vi "HENES_Arduino_Main.vi"() -> ()   [LabVIEW 2023]
uses:
  <vilib>/Instr/_visa.llb/VISA Set IO Buffer Mask.ctl
  <vilib>/Instr/_visa.llb/VISA Flush IO Buffer Mask.ctl
  <vilib>/Platform/TimedLoop/XDataNode/timing_clust.ctl
  <vilib>/Platform/TimedLoop/XDataNode/nitl_modes.ctl
  <vilib>/Platform/TimedLoop/XDataNode/wakeup.ctl
  0e367d9d-ada3-461a-9650-c8cddcce4376.vi
  <vilib>/Utility/file.llb/Read Delimited Spreadsheet (DBL).vi
  <vilib>/Utility/file.llb/Write Delimited Spreadsheet (string).vi
  <vilib>/Instr/_visa.llb/VISA Configure Serial Port (Instr).vi
  <vilib>/Analysis/geometry.llb/Point in Polygon (Array).vi
  <vilib>/Platform/TimedLoop/XDataNode/XDataNode.xnode
  <vilib>/Platform/TimedLoop/XDataNode/XDNodeRunTimeDep.lvlib
  <vilib>/Analysis/NI_AAL_Geometry.lvlib
panel:
  out "read buffer":string
  out "Loop Time":u32=102
  out "배열":dbl[](array[numeric])
  in  "탭 컨트롤":enum32{"Main", "GPS", "ETC."}(tab)
  out "강제 변환(x)":i16
  in  "링":u16(ring) items=["정사각형ROI", "삼각형ROI"]
  in  "ROI_Y":i32=800
  in  "ROI_X":i32=200
  in  "격자크기":dbl=20.0
  out "GO?":bool
  out "Steer_CMD(Deg)":dbl
  out "UTM X(E) INS":dbl format="%#_13g"
  out "UTM Y(N) INS":dbl format="%#_13g"
  out "Near Point":i32
  out "Tracking_Err(m)":dbl
  in  "HLV_Gear":u8
  in  "HLV_A/M":bool
  in  "Input_Spd(kph)":dbl
  out "Remote_M/A":bool
  out "E-STOP":bool
  in  "Map Refresh":bool
  in  "RDDF":path=path "경로를 입력하세요."
  out "Steer_Feed":dbl
  out "Gear_Feed":u8
  out "XY Graph":T1(graph)
  in  "LOG_Forder":path=path "경로를 입력하세요."
  in  "Data Save On/Off":bool
  in  "COM4":refnum<visa-resource-name>="COM18" caption="GPS_Com."
  in  "COM5":refnum<visa-resource-name>="COM16" caption="HENES_Com."
  out "LiDAR_ROI":cluster{"X좌표":i32[], "Y좌표":i32[]}[](graph)
  in  "COM4 2":refnum<visa-resource-name>="COM16" caption="LiDAR_Com."
  out "Alive_PCU":u8(slide) scale=0.0..254.0
  out "GPS_Speed(kph)":dbl format="%#_g kph"
  out "Speed_Feed(RPM)":dbl format="%#_g rpm"
  out "True_Heading":dbl format="%#_15g"
  out "Evt":dbl
  out "WP_no.":i32
  out "Y_long_path_Full":dbl[](array[numeric])
  out "vel. path":dbl[](array[numeric])
  out "X_lat_path_Full":dbl[](array[numeric])
  out "Path_Evt_arr":dbl[](array[numeric])
  out "Path_Vel_arr":dbl[](array[numeric])
  out "Path_long_arr":dbl[](array[numeric])
  out "Path_lat_arr":dbl[](array[numeric])
  out "Evt.Arr":dbl[](array[numeric])
  out "NMEA_Raw_Data":string
  out "RDDF_Velocity":dbl
  out "Output_Spd_CMD(%)":dbl
  out "Size_init":i32
  out "Output_Spd_CMD(kph)":dbl
  in  "Stop":bool
  # "HENES Autonomous Program"
  # "※ 본 프로그램은 무료 배포 프로그램으로 상업용으로는 사용하지 말 것이며 사용 시 생기는 문제에 대해서 작성자는 책임지지 않습니다."
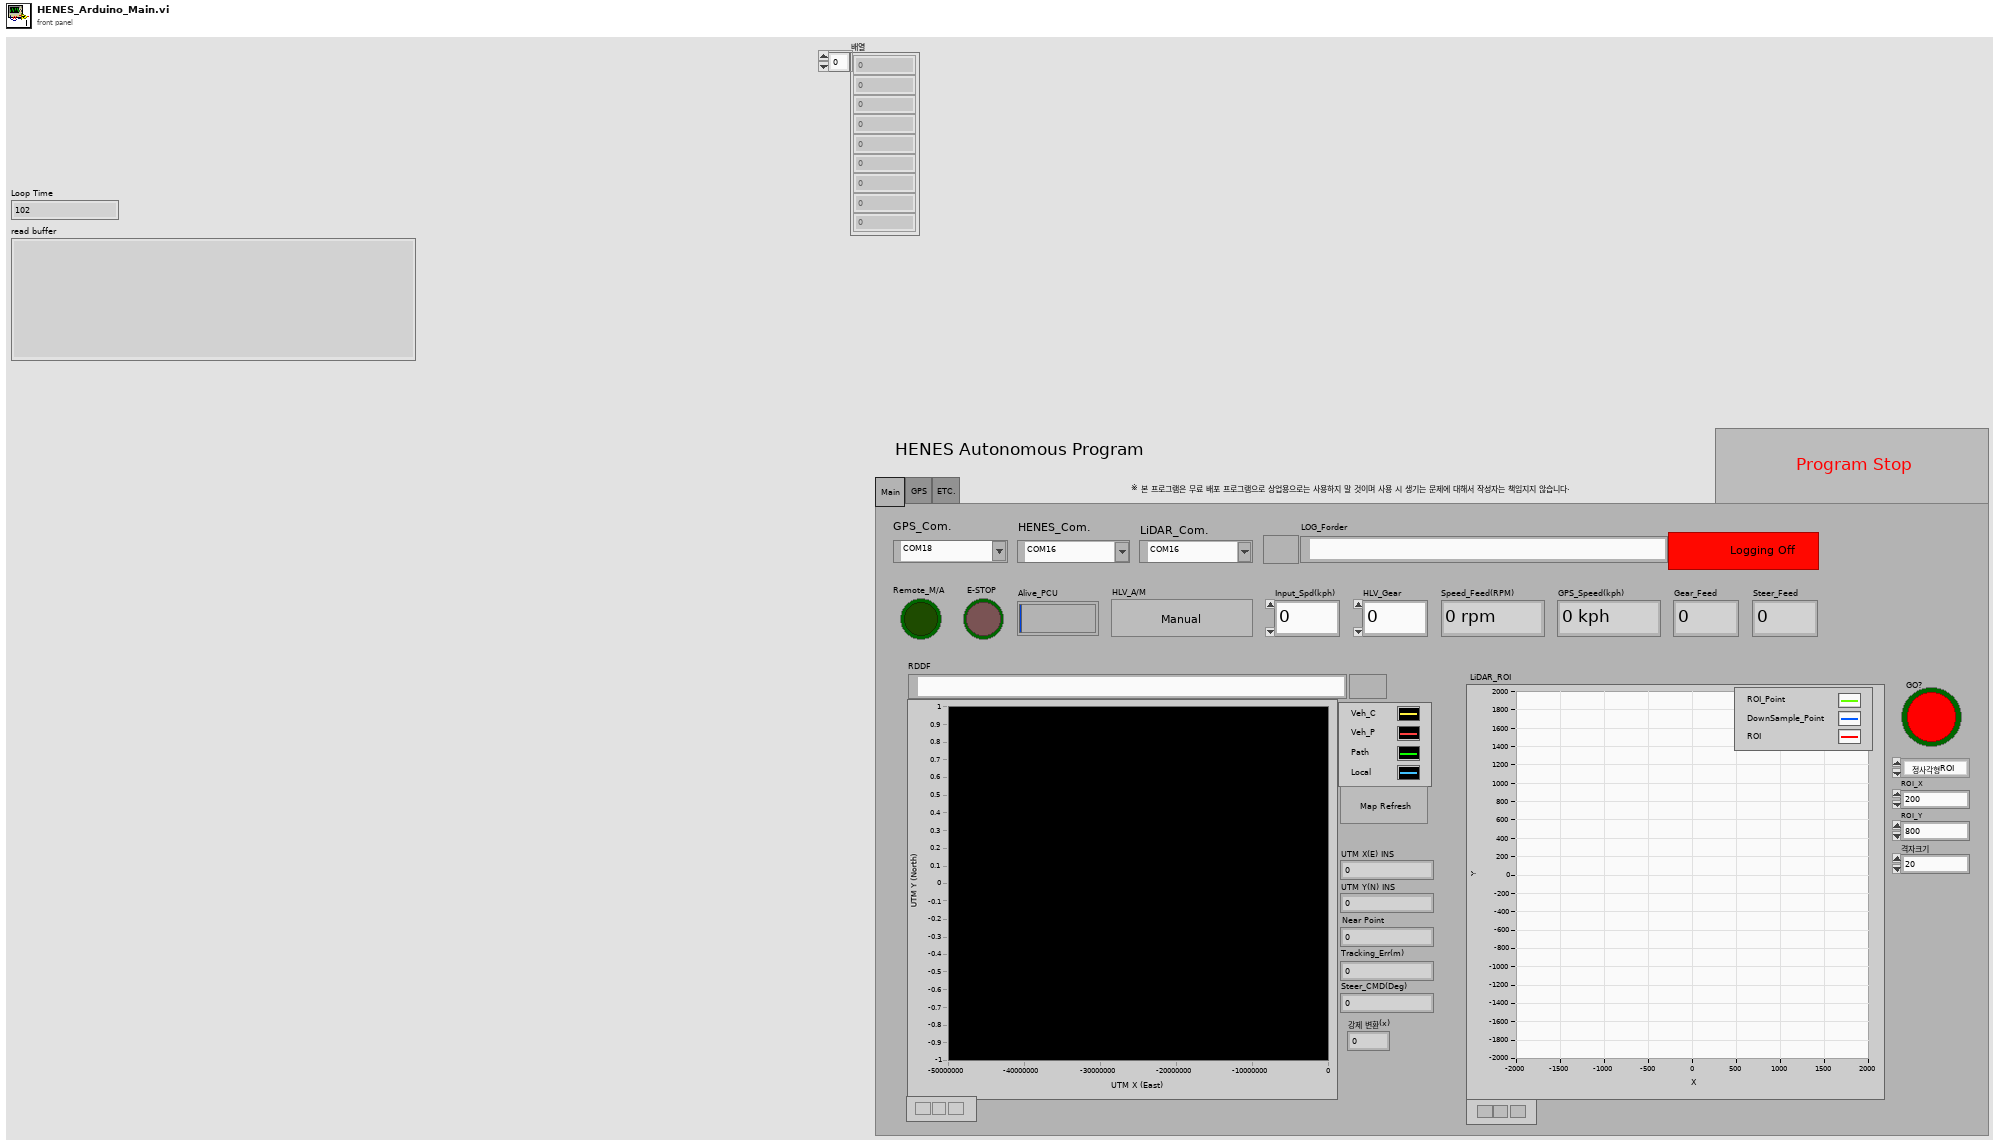
[diagram p1: front panel]
types:
  T1 = cluster{"y_long_path":dbl[], "x_lat_path":dbl[]}[]
  T2 = typedef "VISA Flush IO Buffer Mask.ctl" = u16
  T3 = typedef "VISA Set IO Buffer Mask.ctl" = u16
  T4 = cluster{"HENES_Speed":i16, "HENES_Steer":i16, "HENES_Gear":u8, "HENES_Alive":u8}
  T5 = cluster{"HLV_M/A_Status":u8, "HLV_Speed":i16, "HLV_Steer":i16, "HLV_Gear":u8, "HLV_E-Stop":u8, "HLV_Alive":u8}
  T6 = cluster{"oldest read timestamp":dbl, "latitude (deg)":dbl, "longitude (deg)":dbl, "ground speed (kph)":dbl, "true track angle (deg)":dbl, "altitude above mean sea level (m)":dbl}
  T7 = typedef "NI_AAL_Geometry.lvlib/Point in Polygon Position.ctl" = u16
  T8 = typedef "XDNodeRunTimeDep.lvlib/timing_clust.ctl" = cluster{"Expected End [f-1]":u64, "Actual End [f-1]":u64, "Finished Late? [f-1]":bool, "Expected End [i-1]":u64, "Actual End [i-1]":u64, "Finished Late? [i-1]":bool, "Expected Start [i]":u64, "Actual Start [i]":u64, "Expected Start [f]":u64, "Actual Start [f]":u64, "Source Name":string, "Structure Name":string, "Period":i64, "Deadline":i64, "Offset":i64, "Start":i64, "Priority":i32, "Timeout":i32, "Mode":T9, "Wakeup Reason":T10, "Error":errorcluster, "Source Type":string, "Secondary Source Type":string, "Global End Time":u64, "Global Start Time":u64, "Frame Duration":u64, "Iteration Duration":u64, "Assigned CPU":i32, "I/O Scan Engine Mode":u32}
  T9 = typedef "XDNodeRunTimeDep.lvlib/nitl_modes.ctl" = enum32{"No Change", "Process missed periods, maintain original phase", "Discard missed periods, maintain original phase", "Process missed periods, ignore original phase", "Discard missed periods, ignore original phase"}
  T10 = typedef "XDNodeRunTimeDep.lvlib/wakeup.ctl" = enum32{"Normal", "Aborted", "Asynchronous wakeup", "Timing source error", "Timed loop error", "Timeout"}
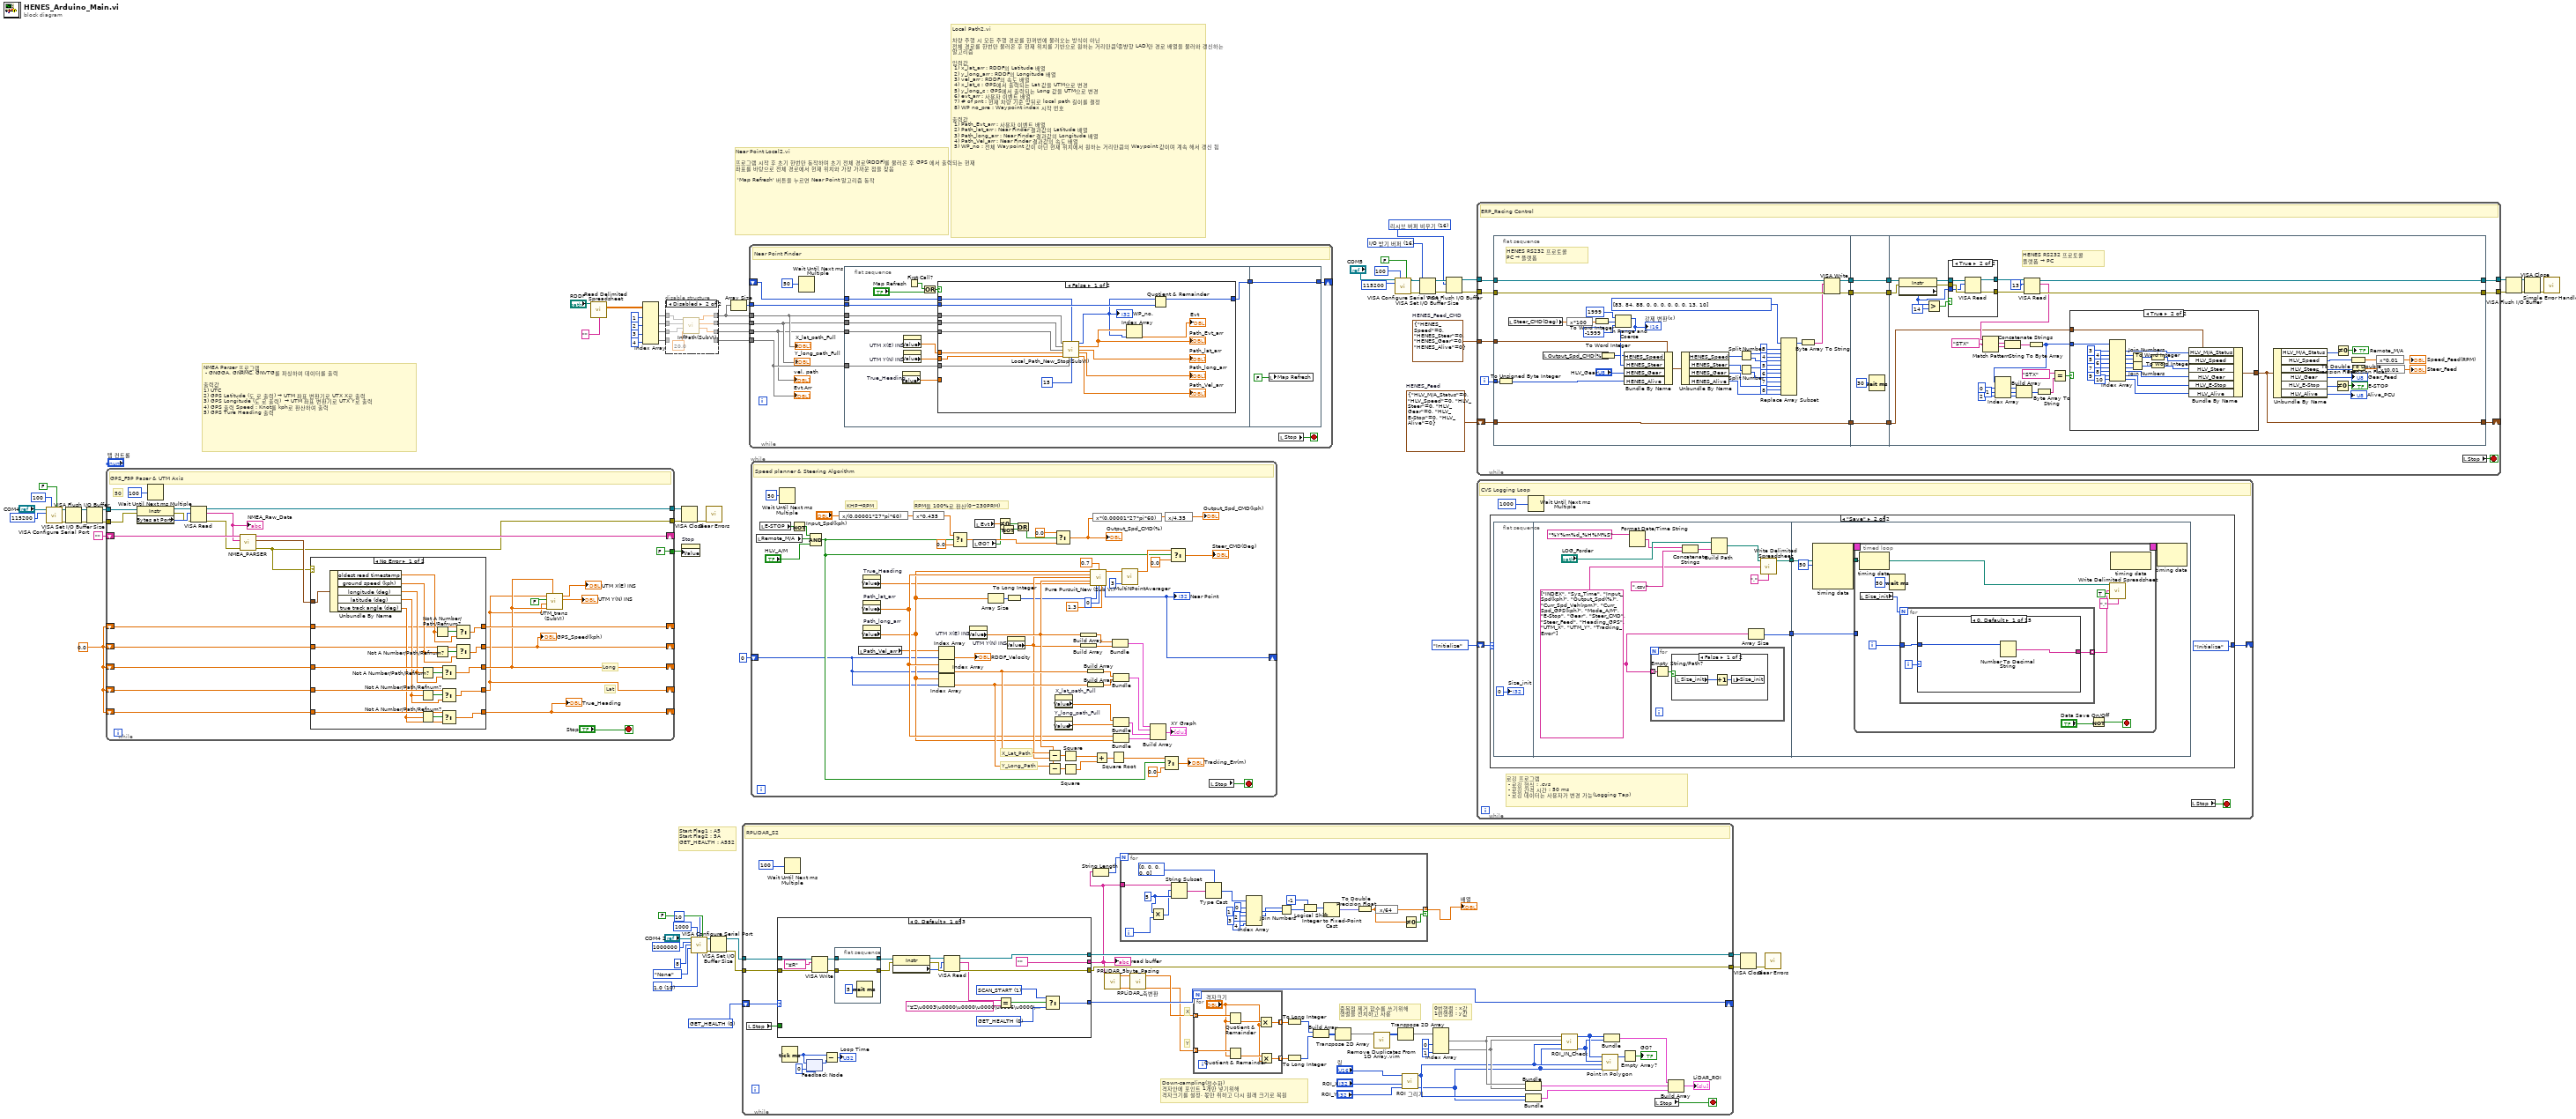
[diagram p0: block diagram]
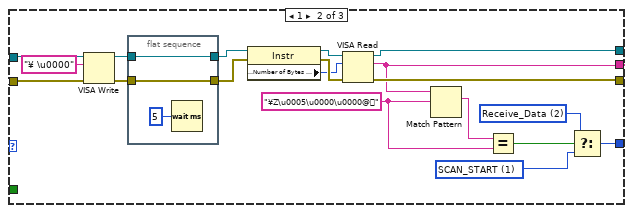
[diagram p2: hidden frame]
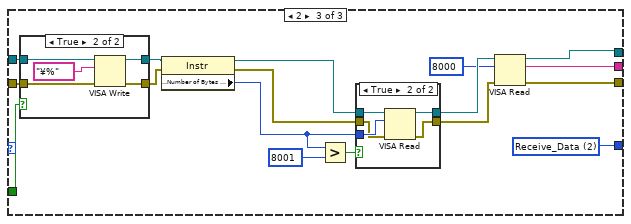
[diagram p3: hidden frame]
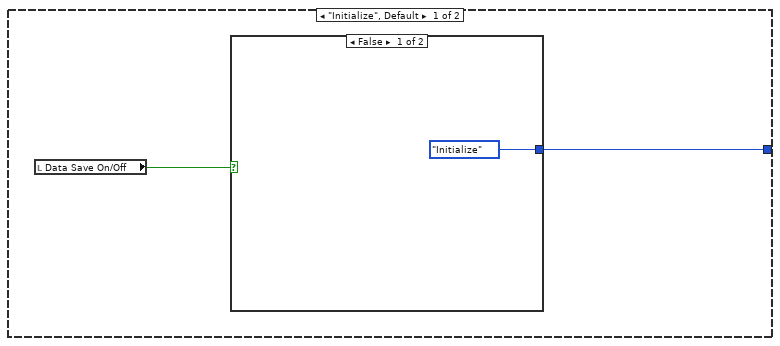
[diagram p6: hidden frame]
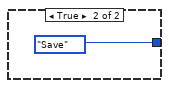
[diagram p7: hidden frame]
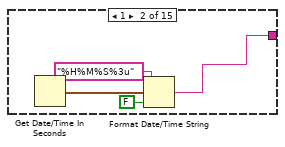
[diagram p9: hidden frame]
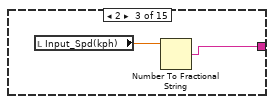
[diagram p10: hidden frame]
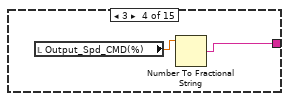
[diagram p11: hidden frame]
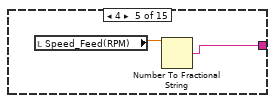
[diagram p12: hidden frame]
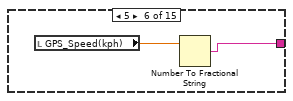
[diagram p13: hidden frame]
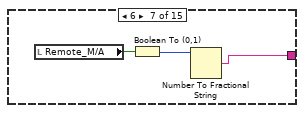
[diagram p14: hidden frame]
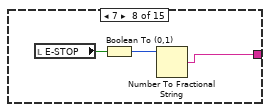
[diagram p15: hidden frame]
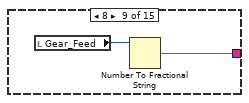
[diagram p16: hidden frame]
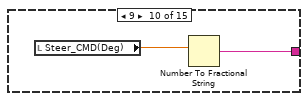
[diagram p17: hidden frame]
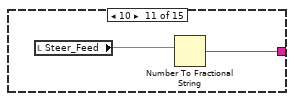
[diagram p18: hidden frame]
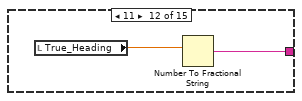
[diagram p19: hidden frame]
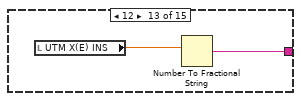
[diagram p20: hidden frame]
diagram:
  w3 = T2 16 items=["리시브 버퍼 비우기"=16, "전달 버퍼 디바이스에 쓰기"=32, "리시브 버퍼 비우기(I/O 없음)"=64, "전달 버퍼 비우기"=128] ("Mask")
  w6 = T3 16 items=["I/O 받기 버퍼"=16, "I/O 전달 버퍼"=32, "I/O 받기와 전달 버퍼"=48] ("Mask")
  w17 = u16 10 items=["1.0"=10, "1.5"=15, "2.0"=20] ("stop bits (10: 1 bit)")
  w19 = u16 0 items=["GET_HEALTH", "SCAN_START", "Receive_Data"]
  w35 = T4 {"HENES_Speed"=0, "HENES_Steer"=0, "HENES_Gear"=0, "HENES_Alive"=0}  # HENES_Feed_CMD
  w34 = T5 {"HLV_M/A_Status"=0, "HLV_Speed"=0, "HLV_Steer"=0, "HLV_Gear"=0, "HLV_E-Stop"=0, "HLV_Alive"=0}  # HENES_Feed
  w54 = 0.0 ("x")
  # "Start Flag1 : A5\nStart Flag2 : 5A \nGET_HEALTH : A552"
  # "NMEA Parser 프로그램\n - GNGGA, GNRMC, GNVTG를 파싱하여 데이터를 출력\n\n출력값 \n1) UTC\n2) GPS Latitude (도 로 출력) → UTM 좌표 변환기로 UTX X로 출력\n3) GPS Longitude (도 로 출력)  → UTM 좌표 변환기로 UTX Y로 출력\n4) GPS 출력 Speed : Knot를 kph로 환산하여 출력\n5) GPS Ture Heading 출력"
  # "Near Point Local2.vi\n\n프로그램 시작 후 초기 한번만 동작하며 초기 전체 경로(RDDF)를 불러온 후 GPS 에서 출력되는 현재 좌표를 바탕으로 전체 경로에서 현재 위치와 가장 가까운 점을 찾음\n\n 'Map Refresh' 버튼을 누르면 Near Point 알고리즘 동작"
  # "Local Path2.vi\n\n차량 주행 시 모든 주행 경로를 한꺼번에 불러오는 방식이 아닌\n전체 경로를 한번만 불러온 후 현재 위치를 기반으로 원하는 거리만큼(종뱡항 LAD)만 경로 배열을 불러와 갱신하는 알고리즘\n\n입력값 \n 1) x_lat_arr : RDDF의 Latitude 배열\n 2) y_long_arr : RDDF의 Longitude 배열\n 3) vel_arr : RDDF의 속도 배열\n 4) x_lat_c : GPS에서 출력되는 Lat 값을 UTM으로 변경\n 5) y_long_c : GPS에서 출력되는 Long 값을 UTM으로 변경\n 6) evt_arr : 사용자 이벤트 배열\n 7) # of pnt : 현재 차량 기준 앞뒤로 local path 길이를 결정\n 8) WP no_pre : Waypoint index 시작 번호\n\n출력값 \n 1) Path_Evt_arr : 사용자 이벤트 배열\n 2) Path_lat_arr : Near Finder 결과값의 Latitude 배열\n 3) Path_long_arr : Near Finder 결과값의 Longitude 배열\n 4) Path_Vel_arr : Near Finder 결과값의 속도 배열\n 5) WP_no : 전체 Waypoint 값이 아닌 현재 위치에서 원하는 거리만큼의 Waypoint 값이며 계속 해서 갱신 됨"
  n1 = call-poly "VISA Configure Serial Port"("VISA resource name"="COM4", "timeout (10sec)"=u32 100, "Enable Termination\nChar (T)"=FALSE ("Enable Termination\nChar (T)"), "baud rate (9600)"=u32 115200) -> ("VISA resource name out"=w14:refnum<visa-resource-name>, "error out"=w13:errorcluster)  [unwired: 10 in]
  n2 = VISA Set I/O Buffer Size(VISA resource name=w14, error in (no error)=w13) -> (VISA resource name out=w59:refnum<visa-resource-name>, error out=w58:errorcluster)  [unwired: 2 in]
  n3 = VISA Flush I/O Buffer(VISA resource name=w59, error in (no error)=w58) -> (VISA resource name out=w57:refnum<visa-resource-name>, error out=w56:errorcluster)  [unwired: 1 in]
  n4 = while {
    tunnel: w57 -> [w95]
    tunnel: w56 -> [w93]
    tunnel: [w97] -> w62
    tunnel: [w85] -> w60
    shift-right: [w86] -> _
    shift-left: "" -> [w90]
    shift-right: [w70] -> _
    shift-left: w54 -> [w84]
    shift-right: [w74] -> _
    shift-left: w54 -> [w83]
    shift-right: [w73] -> _
    shift-left: w54 -> [w82]
    shift-right: [w78] -> _
    shift-left: w54 -> [w81]
    shift-right: [w77] -> _
    shift-left: w54 -> [w80]
    tunnel: [FALSE] -> w53
    stop <- "Stop" stop-if-true
    # "Lat"
    # "Long"
    # "50"
    # "GPS_F9P Paser & UTM Axis"
    n5 = property class="Instr"(reference=w95, error in=w93) -> (reference out=w94:refnum<visa-resource-name>, error out=w92:errorcluster, "Bytes at Port"=w96:u32)
    n6 = Wait Until Next ms Multiple(millisecond multiple=u32 100) -> ()  [unwired: 1 out]
    n7 = VISA Read(VISA resource name=w94, byte count=w96, error in (no error)=w92) -> (VISA resource name out=w97:refnum<visa-resource-name>, read buffer=w89:string, error out=w87:errorcluster)  [unwired: 1 out]
    "NMEA_Raw_Data" <- w89
    n8 = call "NMEA_PARSER.vi"("previous partial sentence"=w90, "sensor data"=w89, "error in (no error)"=w87) -> ("remaining partial sentence"=w86:string, "GPS data"=w88:T6, "error out"=w85:errorcluster)  [unwired: 5 in]
    n9 = case shown="No Error" w85 {
      tunnel: w88 -> [w118 _]
      tunnel: w83 -> [w114 w123]
      tunnel: w82 -> [w113 w122]
      tunnel: w81 -> [w112 w121]
      tunnel: [w108 w123] -> w74
      tunnel: [w107 w122] -> w73
      tunnel: [w106 w121] -> w78
      tunnel: w84 -> [w103 w120]
      tunnel: [w102 w120] -> w70
      tunnel: w80 -> [w99 w119]
      tunnel: [w98 w119] -> w77
      frame No Error {
        n10 = Unbundle By Name(w118) -> ("oldest read timestamp"=w100:dbl, "ground speed (kph)"=w104:dbl, "longitude (deg)"=w111:dbl, "latitude (deg)"=w110:dbl, "true track angle (deg)"=w109:dbl)
        n11 = Not A Number/Path/Refnum?(number/path/refnum=w111) -> (NaN/Path/Refnum?=w117:bool)
        n12 = Not A Number/Path/Refnum?(number/path/refnum=w110) -> (NaN/Path/Refnum?=w116:bool)
        n13 = Not A Number/Path/Refnum?(number/path/refnum=w109) -> (NaN/Path/Refnum?=w115:bool)
        n14 = Not A Number/Path/Refnum?(number/path/refnum=w100) -> (NaN/Path/Refnum?=w101:bool)
        n15 = Not A Number/Path/Refnum?(number/path/refnum=w104) -> (NaN/Path/Refnum?=w105:bool)
        n16 = Select(t=w114, s=w117, f=w111) -> (s? t:f=w108:dbl)
        n17 = Select(t=w113, s=w116, f=w110) -> (s? t:f=w107:dbl)
        n18 = Select(t=w112, s=w115, f=w109) -> (s? t:f=w106:dbl)
        n19 = Select(t=w99, s=w101, f=w100) -> (s? t:f=w98:dbl)
        n20 = Select(t=w103, s=w105, f=w104) -> (s? t:f=w102:dbl)
      }
      frame Error {
        # "Invalid data points."
      }
    }
    "True_Heading" <- w78
    "GPS_Speed(kph)" <- w70
    n21 = call "UTM_trans (SubVI).vi"("Long_Deg"=w74, "long"=w74, "lat"=w73, "East?West?"=FALSE, "Lat_Deg"=w73) -> ("UTM_Y(Northing)"=→"UTM Y(N) INS":dbl, "UTM_X(Easting)"=→"UTM X(E) INS":dbl)  [unwired: 2 out]
  }
  n22 = call-poly <vilib>:"Read Delimited Spreadsheet.vi"("file path (dialog if empty)"="RDDF", "delimiter (\\t)"="" ("delimiter (\\t)")) -> ("all rows"=w64:dbl[][])  [unwired: 8 in, 5 out]
  n23 = Index Array(array=w64, index (col) #1=1 ("비활성화된 인덱스 (열)"), index (col) #2=2 ("인덱스 (열)"), index (col) #3=3 ("인덱스 (열)"), index (col) #4=4 ("인덱스 (열)")) -> (element #1=w43:dbl[], element #2=w42:dbl[], element #3=w41:dbl[], element #4=w40:dbl[])  [unwired: 4 in]
  n24 = disable-structure shown="Disabled" {
    disable-tunnel: w43 -> [w127 w134]
    disable-tunnel: w42 -> [w126 w133]
    disable-tunnel: w41 -> [w125 w132]
    disable-tunnel: w40 -> [w124 _]
    disable-tunnel: [w127 w130] -> w39
    disable-tunnel: [w126 w129] -> w38
    disable-tunnel: [w125 w128] -> w37
    disable-tunnel: [w124 _] -> w36
    frame Enabled {
    }
    frame Disabled {
      n25 = call "InfPath(SubVI).vi"("Mod dist."=20.0, "vel."=w132, "y_long"=w133, "x_lat"=w134) -> ("vel. path"=w128:dbl[], "y_long_path"=w129:dbl[], "x_lat_path"=w130:dbl[])  [unwired: 1 out]
    }
  }
  n26 = VISA Close(VISA resource name=w62, error in (no error)=w60) -> (error out=w61:errorcluster)
  n27 = property on="Stop" class="Bool (strict)"("Value"=w53) -> ()  [unwired: 2 in, 2 out]
  n28 = call-poly "VISA Configure Serial Port"("VISA resource name"="COM4 2", "timeout (10sec)"=u32 1000, "termination char\n(0xA = '\\n' = LF)"=u8 10 ("termination char\n(0xA = '\\n' = LF)"), "Enable Termination\nChar (T)"=FALSE ("Enable Termination\nChar (T)"), "baud rate (9600)"=u32 1000000, "data bits (8)"=u16 8, "parity (0:none)"=enum16{"None", "Odd", "Even", "Mark", "Space"}."None", "stop bits (10: 1 bit)"=w17) -> ("VISA resource name out"=w27:refnum<visa-resource-name>, "error out"=w26:errorcluster)  [unwired: 6 in]
  n29 = call <vilib>:"Clear Errors.vi"("error in (no error)"=w61) -> ()  [unwired: 5 in, 2 out]
  n30 = VISA Set I/O Buffer Size(VISA resource name=w27, error in (no error)=w26) -> (VISA resource name out=w21:refnum<visa-resource-name>, error out=w20:errorcluster)  [unwired: 2 in]
  n31 = Array Size(array=w39) -> (size(s)=w66:i32)
  n32 = while {
    tunnel: [w169] -> w31
    tunnel: [w170] -> w30
    tunnel: w21 -> [w178]
    tunnel: w20 -> [w177]
    shift-right: [w176] -> _
    shift-left: w19 -> [w179]
    stop <- w135 stop-if-true
    # "0번행렬 : x값\n1번행렬 : y값"
    # "중복점 제거 함수를 쓰기위해\n행렬을 전치하고 사용"
    # "Down-sampling(정수화)\n격자안에 포인트 1개만 넣기위해\n격자크기를 설정, 몫만 취하고 다시 원래 크기로 복원"
    # "Y"
    # "X"
    # "RPLIDAR_S2"
    n33 = local read "Stop"() -> (w175:bool)
    n34 = case shown="0, Default" w179 {
      tunnel: w178 -> [w225 w243 w266]
      tunnel: w177 -> [w224 w242 w265]
      tunnel: [w226 w239 w252] -> w176
      tunnel: [w215 w240 w268] -> w170
      tunnel: [w214 w241 w267] -> w169
      tunnel: w175 -> [_ _ w264]
      tunnel: ["" ("read buffer") w237 w263] -> w137
      frame 0, Default {
        w208 = u16 0 items=["GET_HEALTH", "SCAN_START", "Receive_Data"]
        w209 = u16 1 items=["GET_HEALTH", "SCAN_START", "Receive_Data"]
        n35 = VISA Write(VISA resource name=w225, write buffer="¥R", error in (no error)=w224) -> (VISA resource name out=w219:refnum<visa-resource-name>, error out=w218:errorcluster)  [unwired: 1 out]
        n36 = flat-sequence {
          tunnel: w219 -> [w228]
          tunnel: w218 -> [w227]
          tunnel: [w228] -> w217
          tunnel: [w227] -> w216
          frame #0 {
            n37 = Wait (ms)(milliseconds to wait=u32 5 ("대기 시간 (ms)")) -> ()  [unwired: 1 out]
          }
        }
        n38 = property class="Instr"(reference=w217, error in=w216) -> (reference out=w222:refnum<visa-resource-name>, error out=w221:errorcluster, "Serial Settings:Number of Bytes at Serial Port"=w220:u32)
        n39 = VISA Read(VISA resource name=w222, byte count=w220, error in (no error)=w221) -> (VISA resource name out=w214:refnum<visa-resource-name>, read buffer=w211:string, error out=w215:errorcluster)  [unwired: 1 out]
        n40 = Equal?(x=w211, y="¥Z\u0003\u0000\u0000\u0000\u0006\u0000\u0000\u0000") -> (x = y?=w212:bool)
        n41 = Select(t=w209, s=w212, f=w208) -> (s? t:f=w226:u16)
      }
      frame 1 {
        w230 = u16 2 items=["GET_HEALTH", "SCAN_START", "Receive_Data"]
        w231 = u16 1 items=["GET_HEALTH", "SCAN_START", "Receive_Data"]
        w244 = "¥Z\u0005\u0000\u0000@"
        n42 = VISA Write(VISA resource name=w243, write buffer="¥ \u0000", error in (no error)=w242) -> (VISA resource name out=w246:refnum<visa-resource-name>, error out=w247:errorcluster)  [unwired: 1 out]
        n43 = flat-sequence {
          tunnel: w246 -> [w250]
          tunnel: w247 -> [w249]
          tunnel: [w250] -> w233
          tunnel: [w249] -> w232
          frame #0 {
            n44 = Wait (ms)(milliseconds to wait=u32 5 ("대기 시간 (ms)")) -> ()  [unwired: 1 out]
          }
        }
        n45 = property class="Instr"(reference=w233, error in=w232) -> (reference out=w236:refnum<visa-resource-name>, error out=w235:errorcluster, "Serial Settings:Number of Bytes at Serial Port"=w234:u32)
        n46 = VISA Read(VISA resource name=w236, byte count=w234, error in (no error)=w235) -> (VISA resource name out=w241:refnum<visa-resource-name>, read buffer=w237:string, error out=w240:errorcluster)  [unwired: 1 out]
        n47 = Match Pattern(string=w237, regular expression=w244) -> (match substring=w238:string)  [unwired: 1 in, 3 out]
        n48 = Equal?(x=w238, y=w244) -> (x = y?=w248:bool)
        n49 = Select(t=w230, s=w248, f=w231) -> (s? t:f=w239:u16)
      }
      frame 2 {
        w252 = u16 2 items=["GET_HEALTH", "SCAN_START", "Receive_Data"]
        n50 = case shown="True" w264 {
          tunnel: w266 -> [w277 w281]
          tunnel: w265 -> [w276 w280]
          tunnel: [w277 w279] -> w262
          tunnel: [w276 w278] -> w261
          frame False {
          }
          frame True {
            n51 = VISA Write(VISA resource name=w281, write buffer="¥%", error in (no error)=w280) -> (VISA resource name out=w279:refnum<visa-resource-name>, error out=w278:errorcluster)  [unwired: 1 out]
          }
        }
        n52 = property class="Instr"(reference=w262, error in=w261) -> (reference out=w257:refnum<visa-resource-name>, error out=w256:errorcluster, "Serial Settings:Number of Bytes at Serial Port"=w258:u32)
        n53 = Greater?(x=w258, y=u32 8001) -> (0:w260:bool)
        n54 = case shown="True" w260 {
          tunnel: w257 -> [w270 w275]
          tunnel: w258 -> [_ w274]
          tunnel: w256 -> [w269 w273]
          tunnel: [w270 w272] -> w255
          tunnel: [w269 w271] -> w254
          frame False {
          }
          frame True {
            n55 = VISA Read(VISA resource name=w275, byte count=w274, error in (no error)=w273) -> (VISA resource name out=w272:refnum<visa-resource-name>, error out=w271:errorcluster)  [unwired: 2 out]
          }
        }
        n56 = VISA Read(VISA resource name=w255, byte count=u32 8000, error in (no error)=w254) -> (VISA resource name out=w267:refnum<visa-resource-name>, read buffer=w263:string, error out=w268:errorcluster)  [unwired: 1 out]
      }
    }
    "read buffer" <- w137
    n57 = Tick Count (ms)() -> (millisecond timer value=w174:u32)
    n58 = Wait Until Next ms Multiple(millisecond multiple=u32 100 ("ms 배수")) -> ()  [unwired: 1 out]
    n59 = feedback #1(u32 0 ("millisecond timer value")) -> (w173:u32)
    n60 = feedback-in #1(w174) -> ()
    n61 = Subtract(x=w174, y=w173) -> (x-y=→"Loop Time":u32)
    n62 = String Length(string=w137) -> (length=w138:i32)
    n63 = call "PRLIDAR_5byte_Pasing.vi"("RPLIDAR_Data"=w137) -> ("Distance(mm)"=w150:dbl[], "Theta(deg)"=w151:dbl[])  [unwired: 9 in]
    n64 = for {
      N: w138 -> [_]
      tunnel: w137 -> [w200]
      tunnel: [w182] -> w136 mode=indexing if=w180
      i -> [w199]
      w198 = 5
      n65 = Multiply(x=w198, y=w199) -> (x*y=w197:i32)
      n66 = String Subset(string=w200, offset (0)=w197, length (rest)=w198) -> (substring=w196:string)
      n67 = Type Cast(type=u8[] [0, 0, 0, 0, 0], x=w196) -> (*(type *) &x=w194:u8[])
      n68 = Index Array(array=w194, index #1=0 ("인덱스"), index #2=1 ("인덱스"), index #3=2 ("인덱스"), index #4=3 ("인덱스"), index #5=4 ("인덱스")) -> (element #2=w188:u8, element #3=w183:u8)  [unwired: 3 out]
      n69 = Join Numbers(hi=w183, lo=w188) -> ((hi.lo)=w187:u16)
      n70 = Logical Shift(y=i16 -1, x=w187) -> (x << y=w185:u16)
      n71 = Integer to Fixed-Point Cast(integer=w185) -> (fixed-point=w184:fxp<+,16,16>)  [unwired: 1 in]
      n72 = To Double Precision Float(number=w184) -> (double precision float=w181:dbl)
      n73 = expression code="x/64"(w181) -> (w182:dbl)
      n74 = Not Equal To 0?(x=w181) -> (x != 0?=w180:bool)
    }
    "배열" <- w136
    n75 = call "RPLiDAR_축변환.vi"("Distance(mm)"=w150, "Theta(deg)"=w151) -> ("Y"=w148:dbl[], "X"=w149:dbl[])  [unwired: 8 in]
    n76 = for {
      tunnel: w149 -> [w207] mode=indexing
      tunnel: w148 -> [w206] mode=indexing
      tunnel: [w203] -> w167 mode=indexing
      tunnel: [w202] -> w168 mode=indexing
      n77 = Quotient & Remainder(x=w207, y="격자크기") -> (floor(x/y)=w205:dbl)  [unwired: 1 out]
      n78 = Quotient & Remainder(x=w206, y="격자크기") -> (floor(x/y)=w204:dbl)  [unwired: 1 out]
      n79 = Multiply(x=w205, y="격자크기") -> (x*y=w203:dbl)
      n80 = Multiply(x=w204, y="격자크기") -> (x*y=w202:dbl)
    }
    n81 = To Long Integer(number=w167) -> (32bit integer=w161:i32[])
    n82 = To Long Integer(number=w168) -> (32bit integer=w160:i32[])
    n83 = Build Array(w161, w160) -> (w163:i32[][])
    n84 = Transpose 2D Array(2D array=w163) -> (transposed array=w158:i32[][])
    n85 = call "Remove Duplicates From 1D Array.vim"("array"=w158) -> ("array with duplicates removed"=w159:i32[][])  [unwired: 10 in]
    n86 = Transpose 2D Array(2D array=w159) -> (transposed array=w164:i32[][])
    n87 = call "ROI 그리기.vi"("ROI_Y"="ROI_Y", "ROI_X"="ROI_X", "도형형태"="링") -> ("Y좌표"=w141:i32[], "X좌표"=w142:i32[])  [unwired: 7 in]
    n88 = Index Array(array=w164, index (row) #1=0 ("index (row)"), index (row) #2=1 ("index (row)")) -> (element #1=w144:i32[], element #2=w143:i32[])  [unwired: 2 in]
    n89 = Bundle(w144, w143) -> (w155:cluster{i32[], i32[]})  [unwired: 1 in]
    n90 = Bundle("X좌표"=w142, "Y좌표"=w141) -> (w154:cluster{"X좌표":i32[], "Y좌표":i32[]})  [unwired: 1 in]
    n91 = call "ROI_IN_Check.vi"("도형Y좌표"=w141, "도형X좌표"=w142, "LiDAR_Y"=w143, "LiDAR_X"=w144) -> ("ROI_IN_Y"=w139:i32[], "ROI_IN_X"=w140:i32[])  [unwired: 6 in]
    n92 = call-poly <vilib>:"Point in Polygon.vi"("Polygon Y"=w141, "Polygon X"=w142, "Y"=w139, "X"=w140) -> ("Position"=w152:T7[])  [unwired: 6 in, 1 out]
    n93 = Bundle("ROI_IN_X"=w140, "ROI_IN_Y"=w139) -> (w156:cluster{"ROI_IN_X":i32[], "ROI_IN_Y":i32[]})  [unwired: 1 in]
    n94 = Empty Array?(array=w152) -> (empty?=→"GO?":bool)
    n95 = local read "Stop"() -> (w135:bool)
    n96 = Build Array(w156, w155, w154) -> (→"LiDAR_ROI":cluster{"X좌표":i32[], "Y좌표":i32[]}[])
  }
  n97 = while {
    shift-right: [w291] -> _
    shift-left: _ -> [w292]
    tunnel: w66 -> [w289]
    tunnel: w37 -> [w283]
    tunnel: w38 -> [w284]
    tunnel: w39 -> [w285]
    tunnel: w36 -> [w288]
    stop <- w287 stop-if-true
    # "Near Point Finder"
    n98 = Wait Until Next ms Multiple(millisecond multiple=u32 50) -> ()  [unwired: 1 out]
    n99 = flat-sequence {
      tunnel: [w304] -> w290
      tunnel: w292 -> [w305]
      tunnel: w289 -> [w300]
      tunnel: w283 -> [w299]
      tunnel: w284 -> [w298]
      tunnel: w285 -> [w297]
      tunnel: w288 -> [w296]
      tunnel: [w330] -> w291
      tunnel: w290 -> [w330]
      frame #0 {
        n100 = property on="True_Heading" class="DigNum (strict)"() -> ("Value"=w293:dbl)  [unwired: 2 in, 2 out]
        n101 = property on="UTM X(E) INS" class="DigNum (strict)"() -> ("Value"=w295:dbl)  [unwired: 2 in, 2 out]
        n102 = property on="UTM Y(N) INS" class="DigNum (strict)"() -> ("Value"=w294:dbl)  [unwired: 2 in, 2 out]
        n103 = First Call?() -> (First Call?: T/F=w302:bool)
        n104 = Or(x=w302, y="Map Refresh") -> (x .or. y?=w303:bool)
        n105 = case shown="False" w303 {
          tunnel: w297 -> [w317 w328]
          tunnel: w298 -> [w318 w327]
          tunnel: w305 -> [w316 _]
          tunnel: w299 -> [w319 _]
          tunnel: w300 -> [w320 _]
          tunnel: [w321 w325] -> w304
          tunnel: w296 -> [w311 _]
          tunnel: w295 -> [w310 w324]
          tunnel: w294 -> [w309 w323]
          tunnel: w293 -> [_ w322]
          frame False {
            n106 = call "Local_Path_New_Stop(SubVI).vi"("x_lat_arr"=w317, "WP no_pre"=w316, "y_long_arr"=w318, "vel_arr"=w319, "x_lat_c"=w310, "y_long_c"=w309, "evt_arr"=w311, "# of pnt"=15) -> ("INDEX(Near Point)"=w307:i32, "Evt(Local)"=w313:dbl[], "Lat(Local)"=→"Path_lat_arr":dbl[], "Long(Local)"=→"Path_long_arr":dbl[], "Vel(Local)"=→"Path_Vel_arr":dbl[])  [unwired: 3 in]
            "WP_no." <- w307
            "Path_Evt_arr" <- w313
            n107 = Index Array(array=w313, index=w307) -> (element=→"Evt":dbl)
            n108 = Quotient & Remainder(x=w307, y=w320) -> (x-y*floor(x/y)=w321:i32)  [unwired: 1 out]
          }
          frame True {
            n109 = call "Local_Path_Second (SubVI).vi"("heading_deg"=w322, "heading_limit"=179.0, "y_long"=w323, "x_lat"=w324, "Y_long_path"=w327, "X_lat_path"=w328) -> ("Index(near vehicle)"=w325:i32)  [unwired: 1 out]
          }
        }
      }
      frame #1 {
        n110 = local write "Map Refresh"(FALSE ("Refresh")) -> ()
      }
    }
    n111 = local read "Stop"() -> (w287:bool)
    "X_lat_path_Full" <- w285
    "vel. path" <- w283
    "Y_long_path_Full" <- w284
    "Evt.Arr" <- w288
  }
  n112 = while {
    shift-right: [w375] -> _
    shift-left: 0 -> [w345]
    stop <- w355 stop-if-true
    # "RPM을 100%로 환산(0~230PRM)"
    # "KHP→RPM"
    # "X_Lat_Path"
    # "Y_Long_Path"
    # "Speed planner & Steering Algorithm"
    n113 = local read "Remote_M/A"() -> (w350:bool)
    n114 = local read "E-STOP"() -> (w346:bool)
    n115 = Wait Until Next ms Multiple(millisecond multiple=u32 50 ("ms 배수")) -> ()  [unwired: 1 out]
    n116 = Not(x=w346) -> (.not. x?=w347:bool)
    n117 = Compound Arithmetic op=AND ("복합 연산")(w347, w350, "HLV_A/M") -> (w348:bool)
    n118 = expression code="x/(0.00001*27*pi*60)"("Input_Spd(kph)") -> (w340:dbl)
    n119 = local read "Path_Vel_arr"() -> (w344:dbl[])
    n120 = property on="True_Heading" class="DigNum (strict)"() -> ("Value"=w356:dbl)  [unwired: 2 in, 2 out]
    n121 = property on="Path_lat_arr" class="Arr (strict)"() -> ("Value"=w369:dbl[])  [unwired: 2 in, 2 out]
    n122 = property on="Path_long_arr" class="Arr (strict)"() -> ("Value"=w368:dbl[])  [unwired: 2 in, 2 out]
    n123 = expression code="x*0.435"(w340) -> (w338:dbl)
    n124 = Index Array(array=w344, index=w345) -> (element=→"RDDF_Velocity":dbl)
    n125 = Index Array(array=w369, index=w345) -> (element=w384:dbl)
    n126 = Index Array(array=w368, index=w345) -> (element=w383:dbl)
    n127 = Select(t=w338, s=w348, f=0.0) -> (s? t:f=w353:dbl)
    n128 = property on="UTM X(E) INS" class="DigNum (strict)"() -> ("Value"=w373:dbl)  [unwired: 2 in, 2 out]
    n129 = local read "GO?"() -> (w332:bool)
    n130 = local read "Evt"() -> (w363:dbl)
    n131 = Array Size(array=w368) -> (size(s)=w362:i32)
    n132 = Not Equal To 0?(x=w363) -> (x != 0?=w334:bool)
    n133 = Not(x=w332) -> (.not. x?=w331:bool)
    n134 = To Long Integer(number=w362) -> (32bit integer=w361:i32)
    n135 = property on="UTM Y(N) INS" class="DigNum (strict)"() -> ("Value"=w372:dbl)  [unwired: 2 in, 2 out]
    n136 = Or(x=w334, y=w331) -> (x .or. y?=w333:bool)
    n137 = Subtract(x=w384, y=w372) -> (x-y=w382:dbl)
    n138 = Subtract(x=w383, y=w373) -> (x-y=w381:dbl)
    n139 = property on="Y_long_path_Full" class="Arr (strict)"() -> ("Value"=w370:dbl[])  [unwired: 2 in, 2 out]
    n140 = Select(t=0.0, s=w333, f=w353) -> (s? t:f=w337:dbl)
    "Output_Spd_CMD(%)" <- w337
    n141 = property on="X_lat_path_Full" class="Arr (strict)"() -> ("Value"=w371:dbl[])  [unwired: 2 in, 2 out]
    n142 = Square(x=w382) -> (x^2=w380:dbl)
    n143 = Square(x=w381) -> (x^2=w379:dbl)
    n144 = Build Array(w373) -> (w391:dbl[])
    n145 = Build Array(w372) -> (w390:dbl[])
    n146 = Build Array(w384) -> (w389:dbl[])
    n147 = Build Array(w383) -> (w388:dbl[])
    n148 = call "Pure Pursuit_New (Sub VI).vi"("x_lat_path"=w368, "L"=0.7, "y_long_path"=w369, "X_Current"=w372, "Y_Current"=w373, "Heading_Current"=w356, "#pnt"=w361, "WP no_pre"=0, "LAD"=1.3) -> ("Steer_CMD(Deg)"=w357:dbl, "Index(near vehicle)"=w375:i32)  [unwired: 3 in, 2 out]
    "Near Point" <- w375
    n149 = expression code="x*(0.00001*27*pi*60)"(w337) -> (w339:dbl)
    n150 = Add(x=w380, y=w379) -> (x+y=w378:dbl)
    n151 = Square Root(x=w378) -> (sqrt(x)=w367:dbl)
    n152 = Bundle(w391, w390) -> (w385:cluster{dbl[], dbl[]})  [unwired: 1 in]
    n153 = Bundle(w389, w388) -> (w377:cluster{dbl[], dbl[]})  [unwired: 1 in]
    n154 = Bundle("Value"=w371, "Value"=w370) -> (w386:cluster{"Value":dbl[], "Value":dbl[]})  [unwired: 1 in]
    n155 = Bundle("Value"=w369, "Value"=w368) -> (w376:cluster{"Value":dbl[], "Value":dbl[]})  [unwired: 1 in]
    n156 = call "MultiNPointAverager.vi"("N point average"=3 ("WP no_pre"), "Data_input"=w357) -> ("숫자형"=w352:dbl)  [unwired: 9 in]
    n157 = Build Array(w385, w377, w386, w376) -> (→"XY Graph":cluster{"Value":dbl[], "Value":dbl[]}[])
    n158 = Select(t=w367, s=w348, f=0.0) -> (s? t:f=→"Tracking_Err(m)":dbl)
    n159 = expression code="x/4.35"(w339) -> (→"Output_Spd_CMD(kph)":dbl)
    n160 = Select(t=w352, s=w348, f=0.0) -> (s? t:f=→"Steer_CMD(Deg)":dbl)
    n161 = local read "Stop"() -> (w355:bool)
  }
  n162 = call-poly "VISA Configure Serial Port"("VISA resource name"="COM5", "timeout (10sec)"=u32 100, "Enable Termination\nChar (T)"=FALSE ("Enable Termination\nChar (T)"), "baud rate (9600)"=u32 115200) -> ("VISA resource name out"=w2:refnum<visa-resource-name>, "error out"=w1:errorcluster)  [unwired: 10 in]
  n163 = VISA Set I/O Buffer Size(VISA resource name=w2, mask (16)=w6, error in (no error)=w1) -> (VISA resource name out=w5:refnum<visa-resource-name>, error out=w4:errorcluster)  [unwired: 1 in]
  n164 = VISA Flush I/O Buffer(VISA resource name=w5, mask (16)=w3, error in (no error)=w4) -> (VISA resource name out=w50:refnum<visa-resource-name>, error out=w49:errorcluster)
  n165 = while {
    shift-right: [w392] -> _
    shift-left: enum16{"Initialize", "Save"}."Initialize" -> [w393]
    stop <- w395 stop-if-true
    # "로깅 프로그램\n - 로깅 형식 : .cvs\n - 로깅 간격 시간 : 50 ms\n - 로깅 데이터는 사용자가 변경 가능(Logging Tap)"
    # "CVS Logging Loop"
    n166 = case shown="\"Save\"" w393 {
      tunnel: [w396 enum16{"Initialize", "Save"}."Initialize"] -> w392
      frame "Initialize", Default {
        n167 = local read "Data Save On/Off"() -> (w397:bool)
        n168 = case shown="False" w397 {
          tunnel: [enum16{"Initialize", "Save"}."Initialize" enum16{"Initialize", "Save"}."Save"] -> w396
          frame False {
          }
          frame True {
          }
        }
      }
      frame "Save" {
        n169 = flat-sequence {
          tunnel: [w412] -> w402
          tunnel: [w411] -> w401
          tunnel: w402 -> [w422]
          tunnel: w401 -> [w421]
          frame #0 {
            "Size_init" <- 0 ("Size_init")
          }
          frame #1 {
            w404 = string[] ["INDEX", "Sys_Time", "Input_Spd(kph)", "Output_Spd(%)", "Curr_Spd_Veh(rpm)", "Curr_Spd_GPS(kph)", "Mode_A/M", "E-Stop", "Gear", "Steer_CMD", "Steer_Feed", "Heading_GPS", "UTM_X", "UTM_Y", "Tracking_Error"] ("배열")
            n170 = Format Date/Time String(time format string (%c)="%Y%m%d_%H%M%S" ("시간 포맷 문자열 (%c)")) -> (date/time string=w407:string)  [unwired: 2 in]
            n171 = for {
              tunnel: w404 -> [w415] mode=indexing
              n172 = Empty String/Path?(string/path=w415) -> (empty?=w414:bool)
              n173 = case shown="False" w414 {
                frame False {
                  n174 = local read "Size_init"() -> (w417:i32)
                  n175 = Increment(x=w417) -> (x+1=w416:i32)
                  n176 = local write "Size_init"(w416) -> ()
                }
                frame True {
                }
              }
            }
            n177 = Concatenate Strings(w407, ".csv" ("string")) -> (w406:string)
            n178 = Build Path(base path="LOG_Forder", name or relative path=w406) -> (appended path=w408:path)
            n179 = Array Size(array=w404) -> (size(s)=w411:i32)
            n180 = call-poly <vilib>:"Write Delimited Spreadsheet.vi"("file path (dialog if empty)"=w408, "1D data"=w404, "delimiter (\\t)"="," ("delimiter (\\t)")) -> ("new file path (Not A Path if cancelled)"=w412:path)  [unwired: 11 in, 1 out]
          }
          frame #2 {
            n181 = node-c288(i64 50 ("Period")) -> (w420:T8)  [unwired: 3 in]
            n182 = timed-loop {
              tunnel: w422 -> [w431]
              tunnel: w421 -> [_]
              timing: w420 -> [_]
              timing-out: [_] -> w419
              i -> [w429]
              stop <- w424 stop-if-true
              n183 = node-c288() -> ()  [unwired: 1 in, 1 out]
              n184 = local read "Size_init"() -> (w426:i32)
              n185 = Wait (ms)(milliseconds to wait=u32 50) -> ()  [unwired: 1 out]
              n186 = for {
                N: w426 -> [_]
                tunnel: w429 -> [w435]
                tunnel: [w434] -> w428 mode=indexing
                i -> [w436]
                n187 = case shown="0, Default" w436 {
                  tunnel: w435 -> [w438 _ _ _ _ _ _ _ _ _ _ _ _ _ _]
                  tunnel: [w437 w439 w444 w446 w448 w450 w453 w456 w457 w459 w461 w463 w465 w468 w470] -> w434
                  frame 0, Default {
                    n188 = Number To Decimal String(number=w438) -> (decimal integer string=w437:string)  [unwired: 1 in]
                  }
                  frame 1 {
                    n189 = Get Date/Time In Seconds() -> (seconds since 1Jan1904=w441:timestamp)
                    n190 = Format Date/Time String(time format string (%c)="%H%M%S%3u", seconds (now)=w441, UTC format=FALSE) -> (date/time string=w439:string)
                  }
                  frame 2 {
                    n191 = local read "Input_Spd(kph)"() -> (w443:dbl)
                    n192 = Number To Fractional String(number=w443) -> (F-format string=w444:string)  [unwired: 3 in]
                  }
                  frame 3 {
                    n193 = local read "Output_Spd_CMD(%)"() -> (w445:dbl)
                    n194 = Number To Fractional String(number=w445) -> (F-format string=w446:string)  [unwired: 3 in]
                  }
                  frame 4 {
                    n195 = local read "Speed_Feed(RPM)"() -> (w447:dbl)
                    n196 = Number To Fractional String(number=w447) -> (F-format string=w448:string)  [unwired: 3 in]
                  }
                  frame 5 {
                    n197 = local read "GPS_Speed(kph)"() -> (w449:dbl)
                    n198 = Number To Fractional String(number=w449) -> (F-format string=w450:string)  [unwired: 3 in]
                  }
                  frame 6 {
                    n199 = local read "Remote_M/A"() -> (w451:bool)
                    n200 = Boolean To (0,1)(Boolean=w451) -> (0, 1=w452:i16)
                    n201 = Number To Fractional String(number=w452) -> (F-format string=w453:string)  [unwired: 3 in]
                  }
                  frame 7 {
                    n202 = local read "E-STOP"() -> (w455:bool)
                    n203 = Boolean To (0,1)(Boolean=w455) -> (0, 1=w454:i16)
                    n204 = Number To Fractional String(number=w454) -> (F-format string=w456:string)  [unwired: 3 in]
                  }
                  frame 8 {
                    n205 = local read "Gear_Feed"() -> (w458:u8)
                    n206 = Number To Fractional String(number=w458) -> (F-format string=w457:string)  [unwired: 3 in]
                  }
                  frame 9 {
                    n207 = local read "Steer_CMD(Deg)"() -> (w460:dbl)
                    n208 = Number To Fractional String(number=w460) -> (F-format string=w459:string)  [unwired: 3 in]
                  }
                  frame 10 {
                    n209 = local read "Steer_Feed"() -> (w462:dbl)
                    n210 = Number To Fractional String(number=w462) -> (F-format string=w461:string)  [unwired: 3 in]
                  }
                  frame 11 {
                    n211 = local read "True_Heading"() -> (w464:dbl)
                    n212 = Number To Fractional String(number=w464) -> (F-format string=w463:string)  [unwired: 3 in]
                  }
                  frame 12 {
                    n213 = local read "UTM X(E) INS"() -> (w466:dbl)
                    n214 = Number To Fractional String(number=w466) -> (F-format string=w465:string)  [unwired: 3 in]
                  }
                  frame 13 {
                    n215 = local read "UTM Y(N) INS"() -> (w467:dbl)
                    n216 = Number To Fractional String(number=w467) -> (F-format string=w468:string)  [unwired: 3 in]
                  }
                  frame 14 {
                    n217 = local read "Tracking_Err(m)"() -> (w469:dbl)
                    n218 = Number To Fractional String(number=w469) -> (F-format string=w470:string)  [unwired: 3 in]
                  }
                }
              }
              n219 = Not(x="Data Save On/Off") -> (.not. x?=w424:bool)
              n220 = call-poly <vilib>:"Write Delimited Spreadsheet.vi"("file path (dialog if empty)"=w431, "1D data"=w428, "append to file? (new file:F)"=TRUE, "delimiter (\\t)"="," ("delimiter (\\t)")) -> ()  [unwired: 10 in, 2 out]
              n221 = node-c288() -> ()  [unwired: 1 in, 1 out]
            }
            n222 = node-c288(w419) -> ()  [unwired: 1 out]
          }
        }
      }
    }
    n223 = Wait Until Next ms Multiple(millisecond multiple=u32 1000) -> ()  [unwired: 1 out]
    n224 = local read "Stop"() -> (w395:bool)
  }
  n225 = while {
    tunnel: w50 -> [w489]
    tunnel: w49 -> [w488]
    tunnel: [w482] -> w48
    tunnel: [w481] -> w47
    shift-right: [w475] -> _
    shift-left: w34 -> [w479]
    tunnel: w35 -> [w477]
    i -> [w483]
    stop <- w476 stop-if-true
    # "ERP_Racing Control"
    n226 = flat-sequence {
      tunnel: [w522] -> w486
      tunnel: [w521] -> w484
      tunnel: w489 -> [w524]
      tunnel: w488 -> [w523]
      tunnel: w483 -> [w520]
      tunnel: [w519] -> w480
      tunnel: w479 -> [w519]
      tunnel: w477 -> [w518]
      tunnel: [w528] -> w487
      tunnel: w486 -> [w528]
      tunnel: [w527] -> w485
      tunnel: w484 -> [w527]
      tunnel: w480 -> [w525]
      tunnel: [w525] -> w478
      tunnel: w487 -> [w552]
      tunnel: w485 -> [w551]
      tunnel: [w569] -> w482
      tunnel: [w568] -> w481
      tunnel: w478 -> [w539]
      tunnel: [w537] -> w475
      frame #0 {
        # "HENES RS232 프로토콜\nPC → 플랫폼"
        n227 = To Unsigned Byte Integer(number=w520) -> (unsigned 8bit integer=w504:u8)
        n228 = local read "Steer_CMD(Deg)"() -> (w491:dbl)
        n229 = local read "Output_Spd_CMD(%)"() -> (w496:dbl)
        n230 = expression code="x*100"(w491) -> (w490:dbl)
        n231 = To Word Integer(number=w490) -> (16bit integer=w494:i16)
        n232 = To Word Integer(number=w496) -> (16bit integer=w495:i16)
        n233 = In Range and Coerce(upper limit=i16 1999 ("상위 리미트"), x=w494, lower limit=i16 -1999 ("상위 리미트")) -> (coerced(x)=w497:i16)  [unwired: 1 out]
        "강제 변환(x)" <- w497
        n234 = Bundle By Name(cluster=w518, "HENES_Speed"=w495, "HENES_Steer"=w497, "HENES_Gear"="HLV_Gear", "HENES_Alive"=w504) -> (w511:T4)
        n235 = Unbundle By Name(w511) -> ("HENES_Speed"=w507:i16, "HENES_Steer"=w503:i16, "HENES_Gear"=w500:u8, "HENES_Alive"=w499:u8)
        n236 = Split Number(x=w507) -> (hi(x)=w506:u8, lo(x)=w505:u8)
        n237 = Split Number(x=w503) -> (hi(x)=w502:u8, lo(x)=w501:u8)
        n238 = Replace Array Subset(array=u8[] [83, 84, 88, 0, 0, 0, 0, 0, 0, 13, 10] ("unsigned byte array"), new element #1=w506, index #1=3, new element #2=w505, index #2=4, new element #3=w502, index #3=5, new element #4=w501, index #4=6, new element #5=w500, index #5=7, new element #6=w499, index #6=8) -> (w509:u8[])
        n239 = Byte Array To String(unsigned byte array=w509) -> (string=w508:string)
        n240 = VISA Write(VISA resource name=w524, write buffer=w508, error in (no error)=w523) -> (VISA resource name out=w522:refnum<visa-resource-name>, error out=w521:errorcluster)  [unwired: 1 out]
      }
      frame #1 {
        n241 = Wait (ms)(milliseconds to wait=u32 30 ("대기 시간 (ms)")) -> ()  [unwired: 1 out]
      }
      frame #2 {
        # "HENES RS232 프로토콜\n플랫폼 → PC"
        n242 = property class="Instr"(reference=w552, error in=w551) -> (reference out=w550:refnum<visa-resource-name>, error out=w549:errorcluster, "Serial Settings:Number of Bytes at Serial Port"=w544:u32)
        n243 = Greater?(x=w544, y=u32 14) -> (0:w546:bool)
        n244 = case shown="True" w546 {
          tunnel: w550 -> [w596 w601]
          tunnel: w549 -> [w595 w600]
          tunnel: [w596 w599] -> w548
          tunnel: [w595 w598] -> w547
          tunnel: w544 -> [_ w597]
          frame False {
          }
          frame True {
            n245 = VISA Read(VISA resource name=w601, byte count=w597, error in (no error)=w600) -> (VISA resource name out=w599:refnum<visa-resource-name>, error out=w598:errorcluster)  [unwired: 2 out]
          }
        }
        n246 = VISA Read(VISA resource name=w548, byte count=u32 13, error in (no error)=w547) -> (VISA resource name out=w569:refnum<visa-resource-name>, read buffer=w567:string, error out=w568:errorcluster)  [unwired: 1 out]
        n247 = Match Pattern(string=w567, regular expression="STX") -> (match substring=w564:string, after substring=w565:string)  [unwired: 1 in, 2 out]
        n248 = Concatenate Strings(w564, w565) -> (w563:string)
        n249 = String To Byte Array(string=w563) -> (unsigned byte array=w541:u8[])
        n250 = Index Array(array=w541, index #1=0, index #2=1, index #3=2) -> (element #1=w558:u8, element #2=w557:u8, element #3=w556:u8)
        n251 = Build Array(w558, w557, w556) -> (w555:u8[])
        n252 = Byte Array To String(unsigned byte array=w555) -> (string=w553:string)
        n253 = Equal?(x="STX", y=w553) -> (x = y?=w540:bool)
        n254 = case shown="True" w540 {
          tunnel: w541 -> [_ w594]
          tunnel: [w571 w581] -> w537
          tunnel: w539 -> [w571 w583]
          frame False {
          }
          frame True {
            n255 = Index Array(array=w594, index #1=3, index #2=4, index #3=5, index #4=6, index #5=7, index #6=8, index #7=9, index #8=10) -> (element #1=w582:u8, element #2=w580:u8, element #3=w579:u8, element #4=w576:u8, element #5=w575:u8, element #6=w574:u8, element #7=w573:u8, element #8=w572:u8)
            n256 = Join Numbers(hi=w580, lo=w579) -> ((hi.lo)=w585:u16)
            n257 = Join Numbers(hi=w576, lo=w575) -> ((hi.lo)=w584:u16)
            n258 = To Word Integer(number=w585) -> (16bit integer=w578:i16)
            n259 = To Word Integer(number=w584) -> (16bit integer=w577:i16)
            n260 = Bundle By Name(cluster=w583, "HLV_M/A_Status"=w582, "HLV_Speed"=w578, "HLV_Steer"=w577, "HLV_Gear"=w574, "HLV_E-Stop"=w573, "HLV_Alive"=w572) -> (w581:T5)
          }
        }
        n261 = Unbundle By Name(w537) -> ("HLV_M/A_Status"=w538:u8, "HLV_Speed"=w533:i16, "HLV_Steer"=w532:i16, "HLV_Gear"=→"Gear_Feed":u8, "HLV_E-Stop"=w536:u8, "HLV_Alive"=→"Alive_PCU":u8)
        n262 = Not Equal To 0?(x=w536) -> (x != 0?=→"E-STOP":bool)
        n263 = Not Equal To 0?(x=w538) -> (x != 0?=→"Remote_M/A":bool)
        n264 = To Double Precision Float(number=w533) -> (double precision float=w543:dbl)
        n265 = To Double Precision Float(number=w532) -> (double precision float=w531:dbl)
        n266 = expression code="x*0.01"(w543) -> (→"Speed_Feed(RPM)":dbl)
        n267 = expression code="x*0.01"(w531) -> (→"Steer_Feed":dbl)
      }
    }
    n268 = local read "Stop"() -> (w476:bool)
  }
  n269 = VISA Close(VISA resource name=w31, error in (no error)=w30) -> (error out=w32:errorcluster)
  n270 = call <vilib>:"Clear Errors.vi"("error in (no error)"=w32) -> ()  [unwired: 5 in, 2 out]
  n271 = VISA Flush I/O Buffer(VISA resource name=w48, error in (no error)=w47) -> (VISA resource name out=w51:refnum<visa-resource-name>, error out=w52:errorcluster)  [unwired: 1 in]
  n272 = VISA Close(VISA resource name=w51, error in (no error)=w52) -> (error out=w46:errorcluster)
  n273 = call <vilib>:"Simple Error Handler.vi"("error in (no error)"=w46) -> ()  [unwired: 4 in, 5 out]
